vi "Paro.vi"() -> ()   [LabVIEW 2016]
panel:
  out "x+1":dbl
  in  "Stop Button":bool
  in  "Boolean":bool
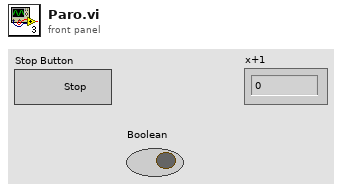
[diagram p1: front panel]
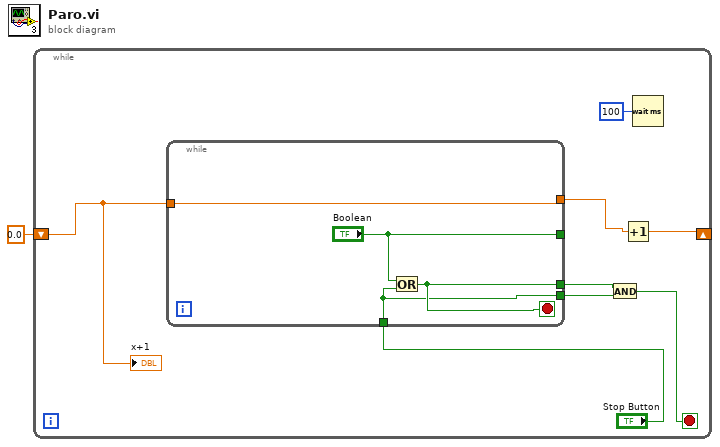
[diagram p0: block diagram]
diagram:
  n1 = while {
    shift-right: [w9] -> _
    shift-left: 0.0 -> [w6]
    stop <- w3 stop-if-true
    n2 = while {
      tunnel: ["Boolean"] -> _
      tunnel: [w13] -> w8
      tunnel: w6 -> [w13]
      tunnel: "Stop Button" -> [w10]
      tunnel: [w11] -> w5
      tunnel: [w10] -> w2
      stop <- w11 stop-if-true
      n3 = Or(x="Boolean", y=w10) -> (x .or. y?=w11:bool)
    }
    n4 = And(x=w5, y=w2) -> (x .and. y?=w3:bool)
    n5 = Increment(x=w8) -> (x+1=w9:dbl)
    n6 = Wait (ms)(milliseconds to wait=u32 100) -> ()  [unwired: 1 out]
    "x+1" <- w6
  }
